vi "Set Bucket Versioning.vi"(7 "Auth Device Data":T1, 8 "error in (no error)":errorcluster, 9 "MFA Delete":T2, 10 "Status":T3, 11 "Bucket in":refnum<class "Bucket.lvclass">) -> (0 "error out":errorcluster, 3 "Bucket out":refnum<class "Bucket.lvclass">)   [LabVIEW 2015, in "NI_AWS_S3.lvlib" / "Bucket.lvclass"]
doc: "This implementation of the PUT operation uses the versioning subresource to set the versioning state of an existing bucket. To set the versioning state, you must be the bucket owner.\n\nYou can set the versioning state with one of the following values:\n\nEnabled—Enables versioning for the objects in the bucket\nAll objects added to the bucket receive a unique version ID.\nSuspended—Disables versioning for the objects in the bucket\nAll objects added to the bucket receive the version ID null.\nIf the versioning state has never been set on a bucket, it has no versioning state; a GET versioning request does not return a versioning state value.\n\nIf the bucket owner enables MFA Delete in the bucket versioning configuration, the bucket owner must include the x-amz-mfa request header and the Status and the MfaDelete request elements in a request to set the versioning state of the bucket.\n\nIf you have an object expiration lifecycle policy in your non-versioned bucket and you want to maintain the same permanent delete behavior when you enable versioning, you must add a noncurrent expiration policy. The noncurrent expiration lifecycle policy will manage the deletes of the noncurrent object versions in the version-enabled bucket. (A version-enabled bucket maintains one current and zero or more noncurrent object versions.) For more information, see Lifecycle and Versioning in the Amazon Simple Storage Service Developer Guide."
uses:
  Bucket.lvclass
  Versioning Status.ctl
  MFA Delete.ctl
  Auth Device Data.ctl
  Core/HTTP Request/Region handling.ctl
  Core/HTTP Request/Request Options.ctl
  Core/HTTP Request/Name Value Pair.ctl
  Core/HTTP Request/URL formatting.ctl
  Bucket.lvclass/Bucket.ctl
  Read Name.vi
  Core/HTTP Request/HTTP Request.lvclass
  NI_AWS_S3.lvlib
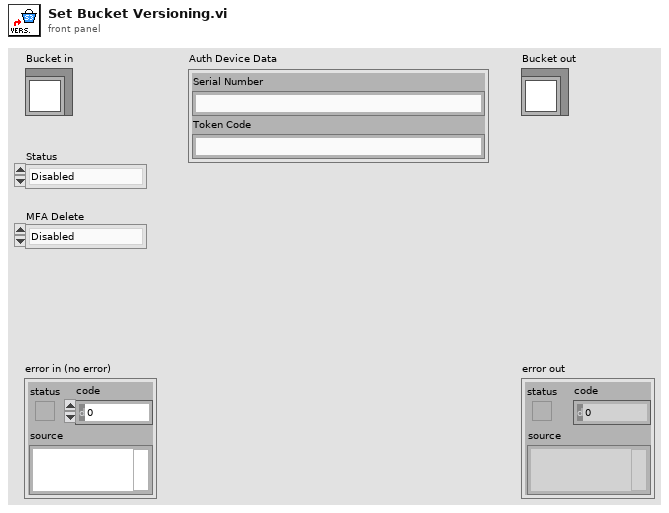
[diagram p1: front panel]
types:
  T1 = typedef "NI_AWS_S3.lvlib/Auth Device Data.ctl" = cluster{"Serial Number":string, "Token Code":string}
  T2 = typedef "NI_AWS_S3.lvlib/MFA Delete.ctl" = enum16{"Disabled", "Enabled"}
  T3 = typedef "NI_AWS_S3.lvlib/Versioning Status.ctl" = enum16{"Disabled", "Suspended", "Enabled"}
  T4 = typedef "NI_AWS_Core.lvlib/HTTP Request.lvclass/Name Value Pair.ctl" = cluster{"name":string, "value":string}
  T5 = typedef "NI_AWS_Core.lvlib/HTTP Request.lvclass/Request Options.ctl" = cluster{"request headers":T4[], "request parameters":T4[], "request body":string, "region handling":T6, "URL formatting":T7}
  T6 = typedef "NI_AWS_Core.lvlib/HTTP Request.lvclass/Region handling.ctl" = enum16{"use region everywhere", "use region (authentication only)", "use region (URL only)", "ignore region everwhere"}
  T7 = typedef "NI_AWS_Core.lvlib/HTTP Request.lvclass/URL formatting.ctl" = enum16{"region-", "region."}
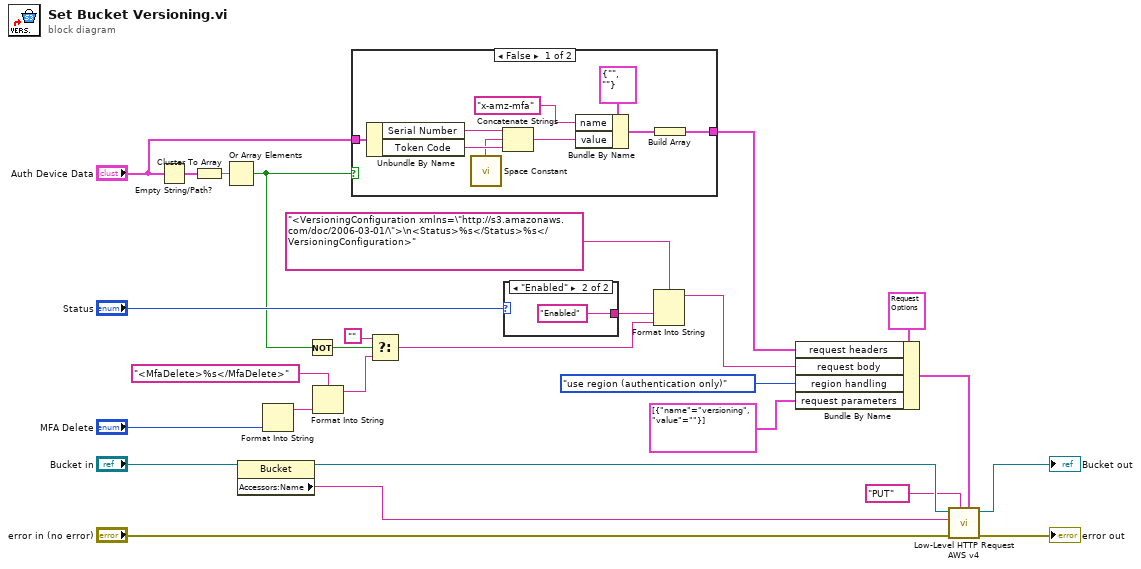
[diagram p0: block diagram]
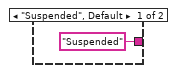
[diagram p3: hidden frame]
diagram:
  n1 = Empty String/Path?(string/path="Auth Device Data") -> (empty?=w10:cluster{"Serial Number":bool, "Token Code":bool})
  n2 = Cluster To Array(cluster=w10) -> (array=w11:bool[])
  n3 = Or Array Elements(Boolean array=w11) -> (logical OR=w8:bool)
  n4 = property class="Bucket"(reference="Bucket in") -> (reference out=w4:refnum<class "Bucket.lvclass">, "Accessors:Name"=w27:string)  [unwired: 1 in, 1 out]
  n5 = Format Into String("MFA Delete") -> (resulting string=w13:string)  [unwired: 3 in, 1 out]
  n6 = Not(x=w8) -> (.not. x?=w5:bool)
  n7 = Format Into String(format string="<MfaDelete>%s</MfaDelete>", w13) -> (resulting string=w12:string)  [unwired: 2 in, 1 out]
  n8 = case shown="False" w8 {
    tunnel: "Auth Device Data" -> [w31 _]
    tunnel: [w29 _] -> w6
    frame False {
      n9 = Unbundle By Name(w31) -> ("Serial Number"=w36:string, "Token Code"=w35:string)
      n10 = call <vilib>:"Space Constant.vi"() -> ("String"=w34:string)
      n11 = Concatenate Strings(w36, w34, w35) -> (w33:string)
      n12 = Bundle By Name(cluster=T4 {"name"="", "value"=""} ("Name Value Pair"), "name"="x-amz-mfa" ("Header"), "value"=w33) -> (w30:T4)
      n13 = Build Array(w30) -> (w29:T4[])
    }
    frame True {
    }
  }
  n14 = Select(t="", s=w5, f=w12) -> (s? t:f=w15:string)
  n15 = case shown="\"Enabled\"" "Status" {
    tunnel: ["Suspended" "Enabled"] -> w16
    frame "Suspended", Default {
    }
    frame "Enabled" {
    }
  }
  n16 = Format Into String(format string="<VersioningConfiguration xmlns=\"http://s3.amazonaws.com/doc/2006-03-01/\">\n<Status>%s</Status>%s</VersioningConfiguration>", w16, w15) -> (resulting string=w7:string)  [unwired: 2 in, 1 out]
  n17 = Bundle By Name(cluster=T5 {"request headers"=[], "request parameters"=[], "request body"="", "region handling"=enum."use region everywhere", "URL formatting"=enum."region."} ("Request Options"), "request headers"=w6, "request body"=w7, "region handling"=Region_handling."use region (authentication only)", "request parameters"=T4[] [{"name"="versioning", "value"=""}]) -> (w2:T5)
  n18 = call "Low-Level HTTP Request AWS v4.vi"("Request Options"=w2, "HTTP-Verb"="PUT", "error in (no error)"="error in (no error)", "URL Prefix"=w27, "AWS Core in"=w4) -> ("error out"=→"error out":errorcluster, "AWS Core out"=→"Bucket out":refnum<class "Bucket.lvclass">)  [unwired: 3 in, 2 out]
